vi "autobroadsidev3.vi"() -> ()   [LabVIEW 2012, in "MainProject.lvrbt"]
uses:
  MainProject.lvrbt
  <vilib>/NXT/HiTechnic/HiTechnic Controls/HiTechnic Port.ctl
  <vilib>/NXT/Block Support/NXT_InputPort.ctl
  <vilib>/NXT/Hardware/Plugins/Tetrix DC Motor/TetrixDCMotorAddress.ctl
  <vilib>/NXT/Hardware/Plugins/Tetrix 180 deg Servo/Tetrix180ServoAddress.ctl
  Drivers/AutoControl3.ctl
  Drivers/AutoDriverControl.ctl
  FTC 2012 - 2013/Controls/SpeedControl.ctl
  <vilib>/NXT/NXTIO Xnodes/NXTIONodeSubVIs/TETRIX IO Check Battery.vi
  <vilib>/NXT/Dual Mode Library/Waits/Wait_Num(msec).vi
  <vilib>/NXT/NXTIO Xnodes/NXTIONodeSubVIs/TETRIX IO Move Servos.vi
  <vilib>/NXT/NXTIO Xnodes/NXTIONodeSubVIs/TETRIX IO Stop DC Motors.vi
  <vilib>/NXT/Dual Mode Library/Sound/Tone.vi
  <vilib>/NXT/Dual Mode Library/Waits/Wait_Num.vi
  <vilib>/NXT/Subs/LVHSConnector.ctl
  <vilib>/NXT/NXTIO Xnodes/AddressXNode/NXTIOAddress.xnode
  <vilib>/NXT/NXTIO Xnodes/NXTIOXNode/NXTIO.xnode
  <vilib>/NXT/LegoClasses/BrickReference/BrickReference.lvclass
panel:
  out "Color":string="Black"
  out "Sector (0-9)":i16
  out "Enabled":bool
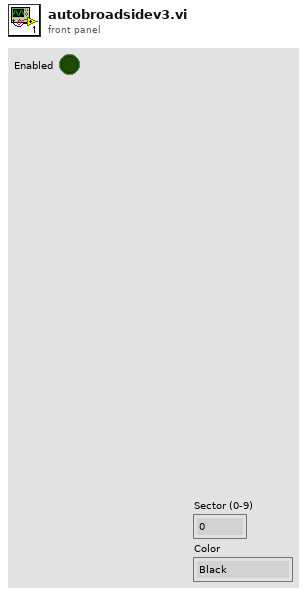
[diagram p1: front panel]
types:
  T1 = typedef "HiTechnic Port.ctl" = cluster{"Port":T2, "MUX Port":u8}
  T2 = typedef "NXT_InputPort.ctl" = u8
  T3 = typedef "TetrixDCMotorAddress.ctl" = i16
  T4 = typedef "LVHSConnector.ctl" = refnum<class "BrickReference.lvclass">
  T5 = typedef "Tetrix180ServoAddress.ctl" = i16
  T6 = typedef "AutoDriverControl.ctl" = enum16{"Init", "Forward", "Reverse", "Left", "Right", "Brake"}
  T7 = typedef "AutoControl3.ctl" = enum16{"FindIRBasket", "DropBLK", "DrvToEndOfBaskets", "DrvAroundBaskets", "AlignWithRamp", "ParkOnRamp", "Stop"}
  T8 = typedef "SpeedControl.ctl" = enum16{"Fast", "Medium", "Slow"}
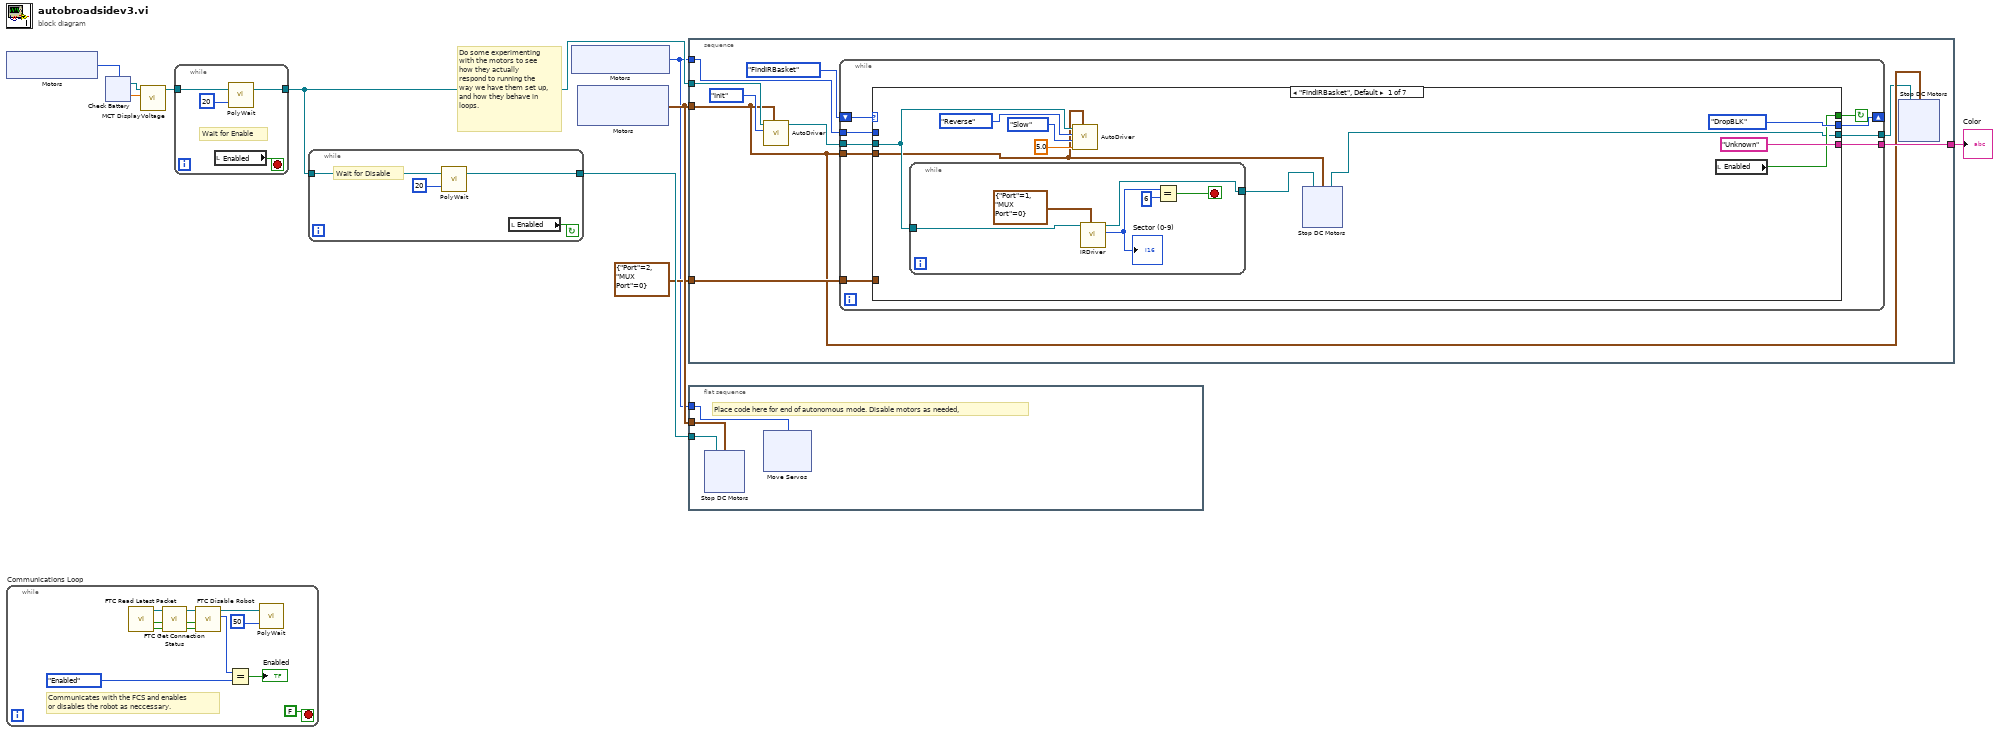
[diagram p0: block diagram]
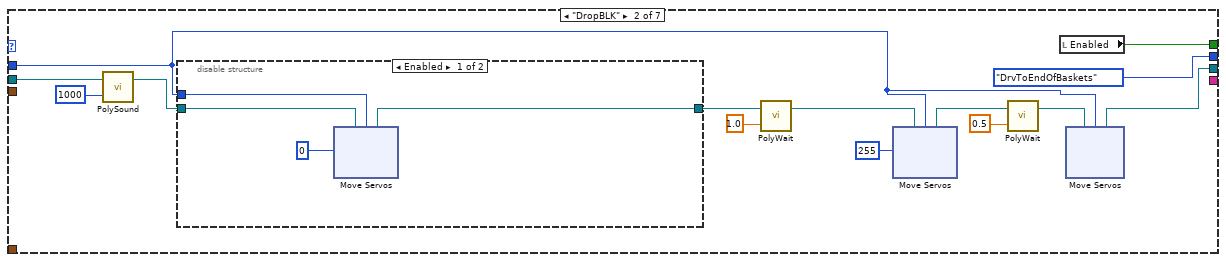
[diagram p2: hidden frame]
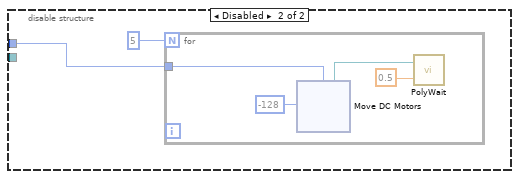
[diagram p3: hidden frame]
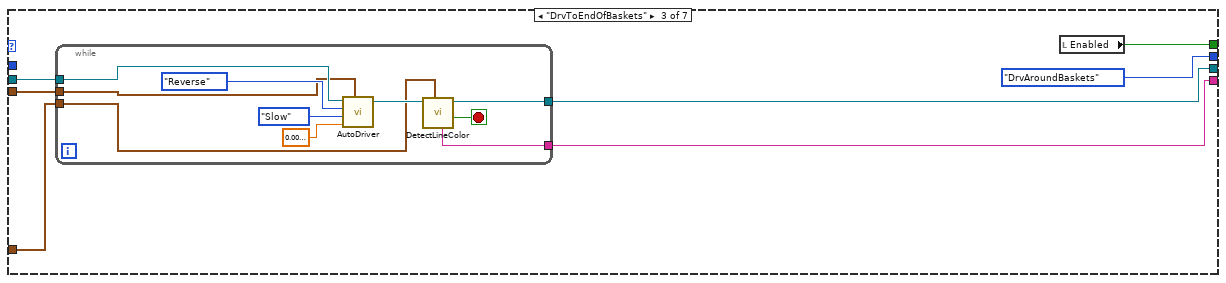
[diagram p4: hidden frame]
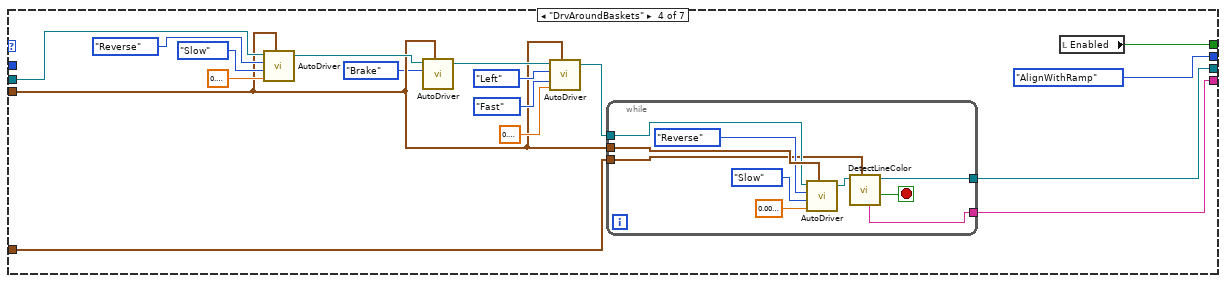
[diagram p5: hidden frame]
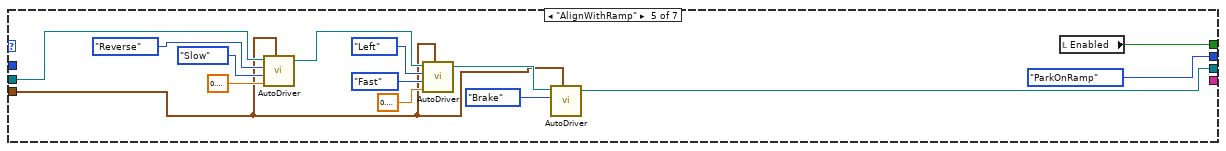
[diagram p6: hidden frame]
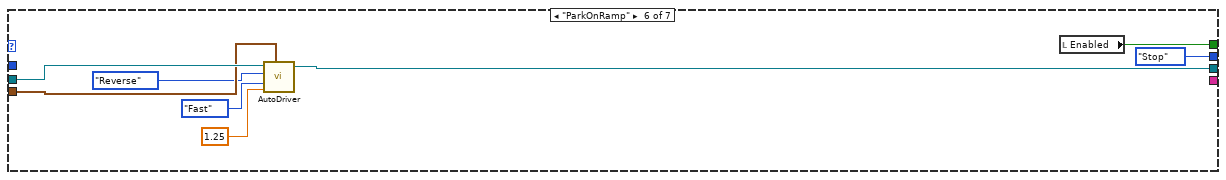
[diagram p7: hidden frame]
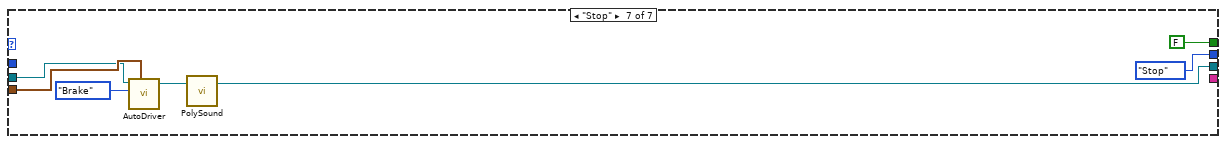
[diagram p8: hidden frame]
diagram:
  # "Do some experimenting with the motors to see how they actually respond to running the way we have them set up, and how they behave in loops."
  n1 = xnode "Motors"() -> ("Motor"=w3:T3)
  n2 = while "Communications Loop" {
    stop <- FALSE stop-if-true
    # "Communicates with the FCS and enables \nor disables the robot as neccessary."
    n3 = call <vilib>:"FTC Read Latest Packet.vi"() -> ("Packet Received?"=w20:bool, "Stopped?"=w19:bool, "NXT"=w22:T4)  [unwired: 6 in, 3 out]
    n4 = call <vilib>:"FTC Get Connection Status.vi"("Packet Received?"=w20, "Stopped?"=w19, "NXT"=w22) -> ("Online?"=w12:bool, "Stopped?"=w13:bool, "NXT"=w21:T4)  [unwired: 5 in]
    n5 = call <vilib>:"FTC Disable Robot.vi"("Online?"=w12, "Stopped?"=w13, "NXT"=w21) -> ("Enabled?"=w15:enum16{"Disabled", "Enabled"}, "NXT"=w17:T4)  [unwired: 3 in]
    n6 = Equal?(x=w15, y=enum16{"Disabled", "Enabled"}."Enabled") -> (x = y?=→"Enabled":bool)
    n7 = call-poly <vilib>:"PolyWait.vi"("Time (100 msec)"=u32 50 ("Time (msec)"), "NXT"=w17) -> ()  [unwired: 2 in, 1 out]
  }
  n8 = xnode "Check Battery"("Motors"=w3) -> ("Voltage 1"=w9:sgl, "NXT"=w10:T4)  [unwired: 1 in]
  n9 = call <vilib>:"MCT DisplayVoltage.vi"("Motor Voltage"=w9, "NXT"=w10) -> ("NXT"=w8:T4)  [unwired: 9 in]
  n10 = while {
    tunnel: [w25] -> w5
    tunnel: w8 -> [w23]
    stop <- w24 stop-if-true
    # "Wait for Enable"
    n11 = local read "Enabled"() -> (w24:bool)
    n12 = call-poly <vilib>:"PolyWait.vi"("Time (100 msec)"=u32 20 ("Time (msec)"), "NXT"=w23) -> ("NXT"=w25:T4)  [unwired: 2 in]
  }
  n13 = while {
    tunnel: [w28] -> w7
    tunnel: w5 -> [w27]
    stop <- w29 continue-if-true
    # "Wait for Disable"
    n14 = call-poly <vilib>:"PolyWait.vi"("Time (100 msec)"=u32 20 ("Time (msec)"), "NXT"=w27) -> ("NXT"=w28:T4)  [unwired: 2 in]
    n15 = local read "Enabled"() -> (w29:bool)
  }
  n16 = xnode "Motors"() -> ("Motor"=w2:T5)
  n17 = xnode "Motors"() -> ("Motor"=w6:cluster{"TetrixDCMotor":T3, "TetrixDCMotor":T3})
  n18 = stacked-sequence {
    tunnel: w6 -> [w32]
    tunnel: w5 -> [w37]
    tunnel: T1 {"Port"=2, "MUX Port"=0} ("Port/MUX") -> [w38]
    tunnel: w2 -> [w34]
    tunnel: [w33] -> w1
    frame #0 {
      n19 = call "AutoDriver.vi"("NXT In"=w37, "Motors"=w32, "Direction"=AutoDriverControl."Init") -> ("NXT Out"=w36:T4)  [unwired: 5 in]
      n20 = while {
        tunnel: w32 -> [w55]
        tunnel: w36 -> [w54]
        shift-right: [w53] -> _
        shift-left: AutoControl3."FindIRBasket" -> [w52]
        tunnel: w38 -> [w51]
        tunnel: w34 -> [w49]
        tunnel: [w48] -> w33
        tunnel: [w47] -> w31
        stop <- w50 continue-if-true
        n21 = case shown="\"FindIRBasket\", Default" w52 {
          tunnel: w55 -> [w60 _ w129 w145 w171 w188 w196]
          tunnel: w54 -> [w61 w81 w130 w157 w177 w189 w195]
          tunnel: [AutoControl3."DropBLK" AutoControl3."DrvToEndOfBaskets" AutoControl3."DrvAroundBaskets" AutoControl3."AlignWithRamp" AutoControl3."ParkOnRamp" AutoControl3."Stop" AutoControl3."Stop"] -> w53
          tunnel: w51 -> [_ _ w127 w149 _ _ _]
          tunnel: [w57 w80 w125 w142 w169 w183 FALSE] -> w50
          tunnel: w49 -> [_ w82 _ _ _ _ _]
          tunnel: ["Unknown" ("Color") _ w126 w143 _ _ _] -> w48
          tunnel: [w56 w79 w124 w141 w168 w182 w190] -> w47
          frame "FindIRBasket", Default {
            n22 = while {
              tunnel: w61 -> [w75]
              tunnel: [w74] -> w58
              stop <- w73 stop-if-true
              n23 = call "IRDriver.vi"("Port"=T1 {"Port"=1, "MUX Port"=0}, "NXT In"=w75) -> ("Sector (0-9)"=w77:i16, "NXT Out"=w74:T4)  [unwired: 8 in]
              "Sector (0-9)" <- w77
              n24 = Equal?(x=w77, y=i16 6) -> (x = y?=w73:bool)
            }
            n25 = call "AutoDriver.vi"("NXT In"=w61, "Motors"=w60, "Direction"=AutoDriverControl."Reverse", "Speed"=SpeedControl."Slow", "Time (1 sec)"=sgl 5.0) -> ()  [unwired: 3 in, 1 out]
            n26 = xnode "Stop DC Motors"("Motors"=w60, "NXT"=w58) -> ("NXT"=w56:T4)
            n27 = local read "Enabled"() -> (w57:bool)
          }
          frame "DropBLK" {
            n28 = call-poly <vilib>:"PolySound.vi"("Duration (500 ms)"=u16 1000, "NXT"=w81) -> ("NXT"=w90:T4)  [unwired: 2 in]
            n29 = disable-structure shown="Enabled" {
              disable-tunnel: w90 -> [w109 _]
              disable-tunnel: w82 -> [w110 w119]
              disable-tunnel: [w107 _] -> w89
              frame Enabled {
                n30 = xnode "Move Servos"("Position 1"=u8 0, "Servos"=w110, "NXT"=w109) -> ("NXT"=w107:T4)
              }
              frame Disabled {
                n31 = for {
                  N: 5 -> [_]
                  tunnel: w119 -> [w122]
                  n32 = xnode "Move DC Motors"("Power/Speed 1"=i8 -128, "Motors"=w122) -> ("NXT"=w121:T4)  [unwired: 1 in]
                  n33 = call-poly <vilib>:"PolyWait.vi"("Time (1 sec)"=sgl 0.5, "NXT"=w121) -> ()  [unwired: 2 in, 1 out]
                }
              }
            }
            n34 = call-poly <vilib>:"PolyWait.vi"("Time (1 sec)"=sgl 1.0, "NXT"=w89) -> ("NXT"=w87:T4)  [unwired: 2 in]
            n35 = xnode "Move Servos"("Position 1"=u8 255, "Servos"=w82, "NXT"=w87) -> ("NXT"=w86:T4)
            n36 = call-poly <vilib>:"PolyWait.vi"("Time (1 sec)"=sgl 0.5, "NXT"=w86) -> ("NXT"=w83:T4)  [unwired: 2 in]
            n37 = local read "Enabled"() -> (w80:bool)
            n38 = xnode "Move Servos"("Servos"=w82, "NXT"=w83) -> ("NXT"=w79:T4)  [unwired: 1 in]
          }
          frame "DrvToEndOfBaskets" {
            n39 = while {
              tunnel: w130 -> [w137]
              tunnel: w129 -> [w136]
              tunnel: w127 -> [w133]
              tunnel: [w132] -> w126
              tunnel: [w131] -> w124
              stop <- w134 stop-if-true
              n40 = call "AutoDriver.vi"("NXT In"=w137, "Motors"=w136, "Direction"=AutoDriverControl."Reverse", "Speed"=SpeedControl."Slow", "Time (1 sec)"=sgl 0.01) -> ("NXT Out"=w135:T4)  [unwired: 3 in]
              n41 = call "DetectLineColor.vi"("Port/MUX"=w133, "NXT In"=w135) -> ("Detected Line?"=w134:bool, "NXT Out"=w131:T4, "Color"=w132:string)  [unwired: 7 in]
            }
            n42 = local read "Enabled"() -> (w125:bool)
          }
          frame "DrvAroundBaskets" {
            n43 = call "AutoDriver.vi"("NXT In"=w157, "Motors"=w145, "Direction"=AutoDriverControl."Reverse", "Speed"=SpeedControl."Slow", "Time (1 sec)"=sgl 0.7) -> ("NXT Out"=w147:T4)  [unwired: 3 in]
            n44 = call "AutoDriver.vi"("NXT In"=w147, "Motors"=w145, "Direction"=AutoDriverControl."Brake") -> ("NXT Out"=w146:T4)  [unwired: 5 in]
            n45 = call "AutoDriver.vi"("NXT In"=w146, "Motors"=w145, "Direction"=AutoDriverControl."Left", "Speed"=SpeedControl."Fast", "Time (1 sec)"=sgl 0.8) -> ("NXT Out"=w150:T4)  [unwired: 3 in]
            n46 = while {
              tunnel: w145 -> [w167]
              tunnel: w150 -> [w166]
              tunnel: w149 -> [w160]
              tunnel: [w159] -> w143
              tunnel: [w158] -> w141
              stop <- w161 stop-if-true
              n47 = call "AutoDriver.vi"("NXT In"=w166, "Motors"=w167, "Direction"=AutoDriverControl."Reverse", "Speed"=SpeedControl."Slow", "Time (1 sec)"=sgl 0.01) -> ("NXT Out"=w162:T4)  [unwired: 3 in]
              n48 = call "DetectLineColor.vi"("Port/MUX"=w160, "NXT In"=w162) -> ("Detected Line?"=w161:bool, "NXT Out"=w158:T4, "Color"=w159:string)  [unwired: 7 in]
            }
            n49 = local read "Enabled"() -> (w142:bool)
          }
          frame "AlignWithRamp" {
            n50 = call "AutoDriver.vi"("NXT In"=w177, "Motors"=w171, "Direction"=AutoDriverControl."Reverse", "Speed"=SpeedControl."Slow", "Time (1 sec)"=sgl 0.3) -> ("NXT Out"=w176:T4)  [unwired: 3 in]
            n51 = call "AutoDriver.vi"("NXT In"=w176, "Motors"=w171, "Direction"=AutoDriverControl."Left", "Speed"=SpeedControl."Fast", "Time (1 sec)"=sgl 0.9) -> ("NXT Out"=w172:T4)  [unwired: 3 in]
            n52 = call "AutoDriver.vi"("NXT In"=w172, "Motors"=w171, "Direction"=AutoDriverControl."Brake") -> ("NXT Out"=w168:T4)  [unwired: 5 in]
            n53 = local read "Enabled"() -> (w169:bool)
          }
          frame "ParkOnRamp" {
            n54 = call "AutoDriver.vi"("NXT In"=w189, "Motors"=w188, "Direction"=AutoDriverControl."Reverse", "Speed"=SpeedControl."Fast", "Time (1 sec)"=sgl 1.25) -> ("NXT Out"=w182:T4)  [unwired: 3 in]
            n55 = local read "Enabled"() -> (w183:bool)
          }
          frame "Stop" {
            n56 = call "AutoDriver.vi"("NXT In"=w195, "Motors"=w196, "Direction"=AutoDriverControl."Brake") -> ("NXT Out"=w193:T4)  [unwired: 5 in]
            n57 = call-poly <vilib>:"PolySound.vi"("NXT"=w193) -> ("NXT"=w190:T4)  [unwired: 3 in]
          }
        }
      }
      n58 = xnode "Stop DC Motors"("Motors"=w32, "NXT"=w31) -> ()  [unwired: 1 out]
    }
  }
  "Color" <- w1
  n59 = flat-sequence {
    tunnel: w7 -> [w199]
    tunnel: w6 -> [w198]
    tunnel: w2 -> [w197]
    frame #0 {
      # "Place code here for end of autonomous mode. Disable motors as needed,"
      n60 = xnode "Stop DC Motors"("Motors"=w198, "NXT"=w199) -> ()  [unwired: 1 out]
      n61 = xnode "Move Servos"("Servos"=w197) -> ()  [unwired: 2 in, 1 out]
    }
  }
